vi "AutoSetDriveParams.vi"(11 "Array":dbl[](array[numeric])) -> (3 "Drive Params":cluster{"Omni":bool, "Low Gear":bool})   [LabVIEW 2013]
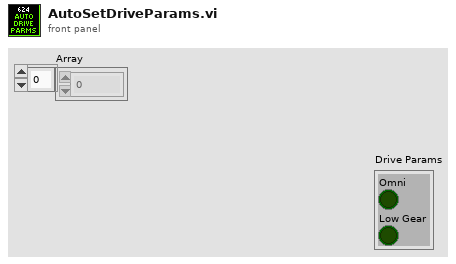
[diagram p1: front panel]
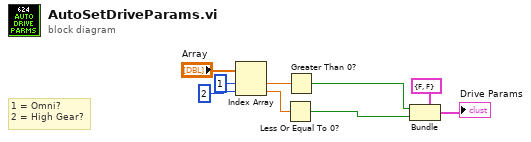
[diagram p0: block diagram]
diagram:
  # "1 = Omni?\n2 = High Gear?"
  n1 = Index Array(array="Array", index #1=1 ("index"), index #2=2 ("index")) -> (element #1=w6:dbl, element #2=w5:dbl)
  n2 = Less Or Equal To 0?(x=w5) -> (x <= 0?=w2:bool)
  n3 = Greater Than 0?(x=w6) -> (x > 0?=w3:bool)
  n4 = Bundle(cluster=cluster{"Omni":bool, "Low Gear":bool} {"Omni"=FALSE, "Low Gear"=FALSE} ("Drive Params 2"), "Omni"=w3, "Low Gear"=w2) -> (→"Drive Params":cluster{"Omni":bool, "Low Gear":bool})
